vi "Test LockinEngine.vi"(8 "error in (no error)":errorcluster, 11 "Lockin.DAQ":refnum<class "Lockin.DAQ.lvclass">) -> (0 "error out":errorcluster, 3 "Lockin.DAQ":refnum<class "Lockin.DAQ.lvclass">)   [LabVIEW 2019, in "Lockin.DAQ.lvclass"]
uses:
  Lockin.DAQ.lvclass
  Typedefs/AO-cluster.ctl
  Instrument.Lockinl.UI/Typedefs/AO Channel--Cluster.ctl
  Typedefs/Function-enum.ctl
  Waveguide Model/Waveguide Model--Cluster.ctl
  Instrument.Lockin/Typedefs/Results Type--Enum.ctl
  Typedefs/Sampling.ctl
  Typedefs/REF-cluster.ctl
  Instrument.Lockinl.UI/Typedefs/REF Channel--Cluster.ctl
  Lockin.DAQ.lvclass/Lockin.DAQ.ctl
  <vilib>/Analysis/baseanly.llb/Mean (DBL).vi
  <vilib>/Analysis/NI_AALBase.lvlib
  Instrument.Lockin/Instrument.Lockin.lvclass
  Instrument.Lockinl.UI/Instrument.Lockin.UI.lvclass
panel:
  in  "Configuration.Channels: REF":T1 {"Order" min=1; "TC" min=0.0001 format="%#_3p"; "Phase" format="%.3g"; "Frequency" min=0.0001 max=10000.0 format="%.3g"}
  out "refresh rate (Hz)":dbl
  out "Waveform Graph":dbl[][](graph)
  in  "buffer size (samples)":i32
  in  "intervals":i32=10
  out "Histogram Graph":T3(graph)
  in  "sampling":T4={"Fs"=204789.0, "#s"=15753}
  in  "Type":T5
  in  "stop":bool
  in  "Simulate Waveguide":bool
  out "Average time (ms)":dbl=0.328125
  in  "Waveguide Cluster":T6
  out "Waveform Chart 2":u32(graph)
  out "Waveform Chart":dbl[][](graph)=[[-0.22911635604378638]]
  in  "AO Chanels":T7=[{"Enable?"=FALSE, "Channel"=0, "Amplitude"=0.0, "Offset"=0.0, "Frequency"=0.1, "Phase"=0.0, "Function"=enum."Sine", "Sweeping?"=FALSE}] {"Phase" format="%.3g"; "Frequency" min=0.0001 max=10000.0 format="%.3g"; "Offset" format="%.3p"; "Amplitude" min=0.0 max=10.0 format="%.3p"}
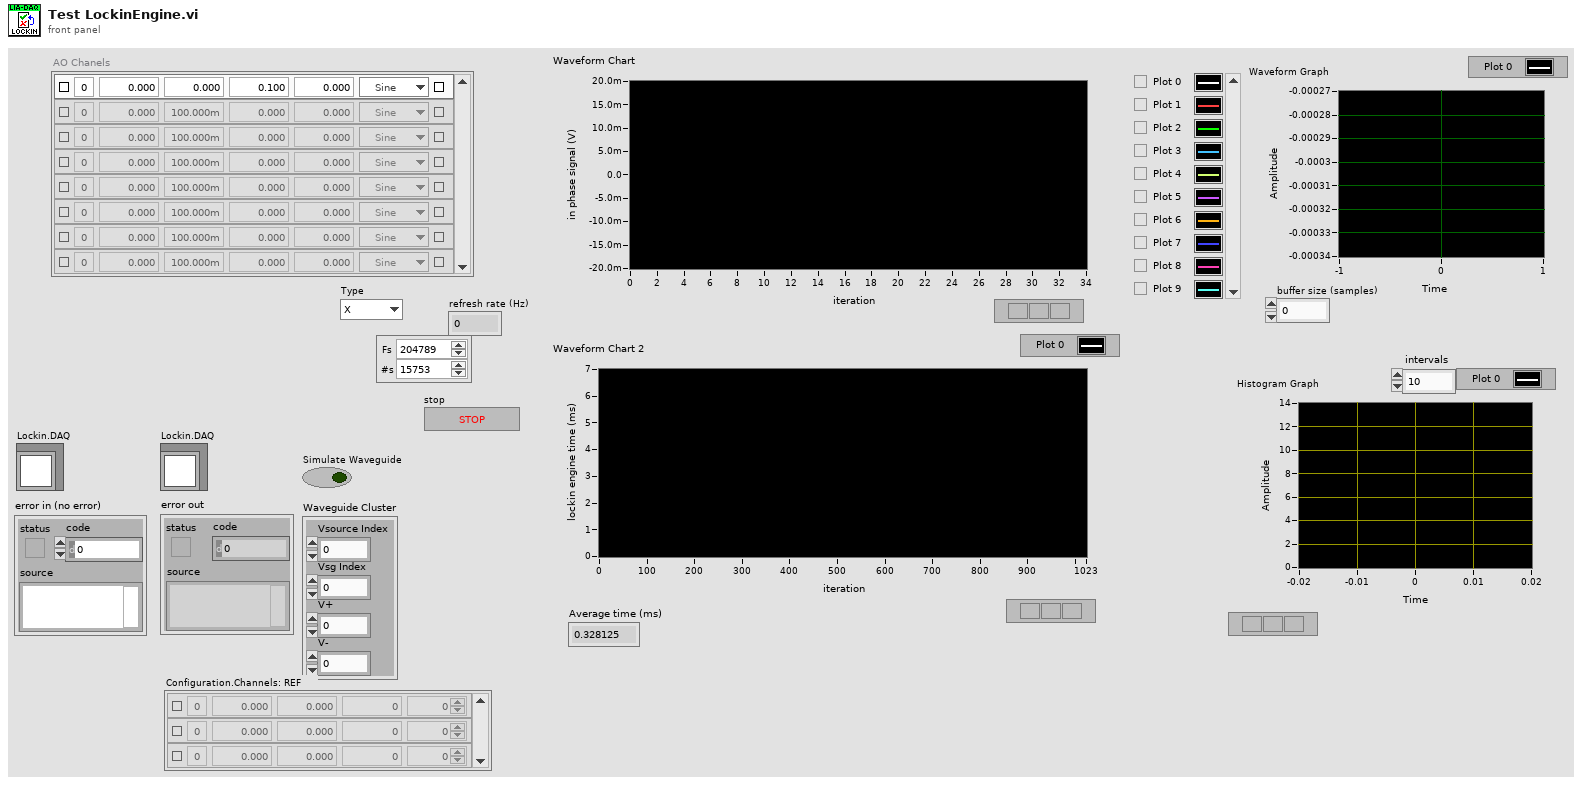
[diagram p1: front panel]
types:
  T1 = typedef "Lockin.DAQ.lvclass/REF-cluster.ctl" = T2[]
  T2 = typedef "Instrument.Lockin.UI.lvclass/REF Channel--Cluster.ctl" = cluster{"Enable?":bool, "Channel":i32, "Frequency":dbl, "Phase":dbl, "TC":dbl, "Order":i32}
  T3 = cluster{"X Values":dbl[], "Histogram: h(x)":i32[]}[]
  T4 = typedef "Lockin.DAQ.lvclass/Sampling.ctl" = cluster{"Fs":dbl, "#s":i32}
  T5 = typedef "Instrument.Lockin.lvclass/Results Type--Enum.ctl" = enum16{"X", "Y", "R", "Theta", "Mean"}
  T6 = typedef "Lockin.DAQ.lvclass/Waveguide Model--Cluster.ctl" = cluster{"Vsource Index":i32, "Vsg Index":i32, "V+":i32, "V-":i32}
  T7 = typedef "Lockin.DAQ.lvclass/AO-cluster.ctl" = T8[]
  T8 = typedef "Instrument.Lockin.UI.lvclass/AO Channel--Cluster.ctl" = cluster{"Enable?":bool, "Channel":i32, "Amplitude":dbl, "Offset":dbl, "Frequency":dbl, "Phase":dbl, "Function":T9, "Sweeping?":bool}
  T9 = typedef "Lockin.DAQ.lvclass/Function-enum.ctl" = enum16{"Sine", "Triangle", "Square"}
  T10 = cluster{"X":waveform(dbl)[], "Y":waveform(dbl)[]}
  T11 = typedef "Lockin.DAQ.lvclass/Results--Cluster.ctl" = cluster{"Time Stamp":timestamp, "Results (Dictionary)":cluster{"key":string, "value":dbl}[]}
  T12 = cluster{"X Values":dbl[], "Histogram: h(x)":i32[]}
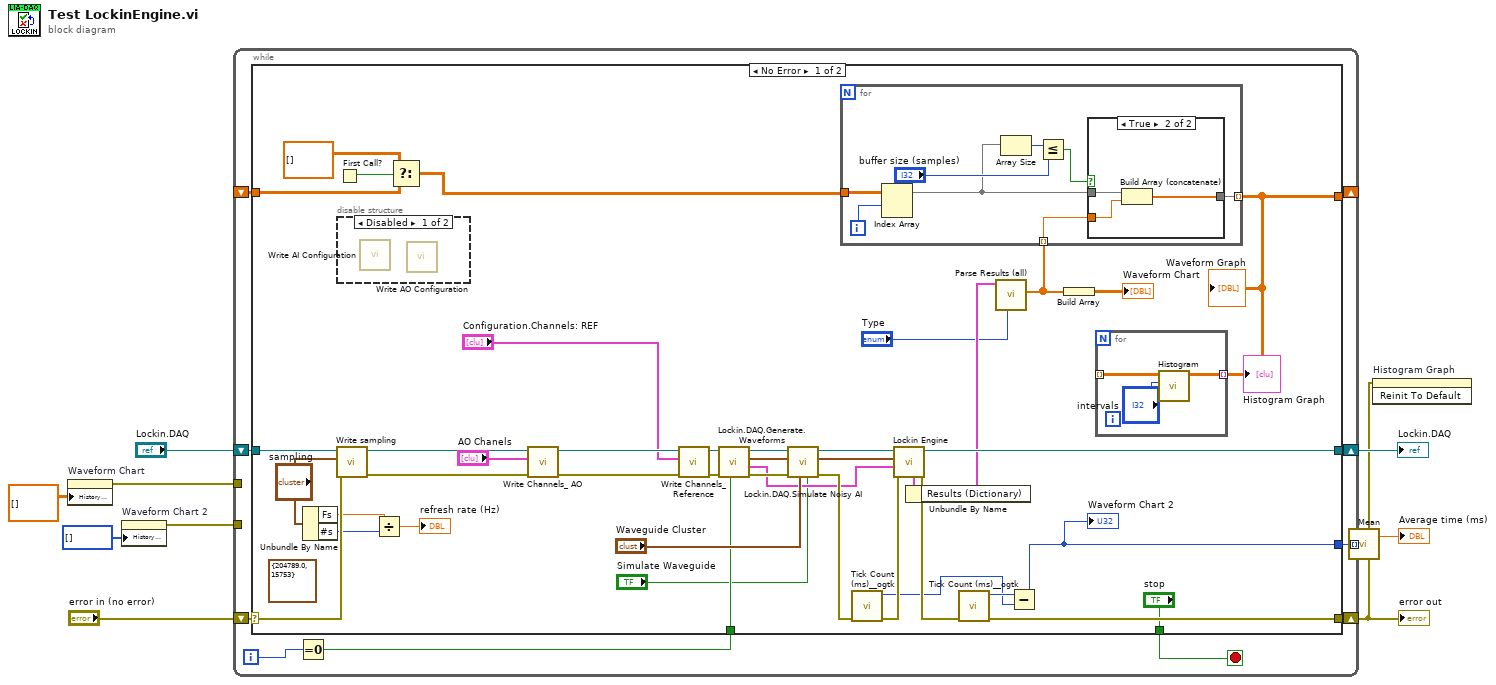
[diagram p0: block diagram]
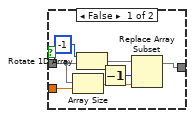
[diagram p2: hidden frame]
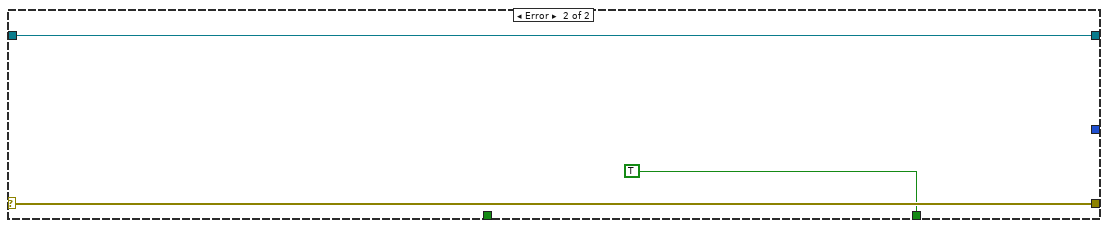
[diagram p4: hidden frame]
diagram:
  n1 = property on="Waveform Chart" class="WFChart (strict)"("History Data"=dbl[][] []) -> (error out=w3:errorcluster)  [unwired: 2 in, 1 out]
  n2 = property on="Waveform Chart 2" class="WFChart (strict)"("History Data"=u32[] []) -> (error out=w4:errorcluster)  [unwired: 2 in, 1 out]
  n3 = while {
    shift-right: [w19] -> w1
    shift-left: "error in (no error)" -> [w20]
    shift-right: [w17] -> w8
    shift-left: "Lockin.DAQ" -> [w18]
    tunnel: [w16] -> w5 mode=indexing
    tunnel: w4 -> [_]
    tunnel: w3 -> [_]
    shift-right: [w12] -> _
    shift-left: _ -> [w11]
    i -> [w14]
    stop <- w13 stop-if-true
    n4 = Equal To 0?(x=w14) -> (x = 0?=w15:bool)
    n5 = case shown="No Error" w20 {
      selector: w20 -> [w59 w87]
      tunnel: [w47 w87] -> w19
      tunnel: [w56 w86] -> w17
      tunnel: w18 -> [w60 w86]
      tunnel: [w45 _] -> w16
      tunnel: w15 -> [w41 _]
      tunnel: ["stop" TRUE ("stop")] -> w13
      tunnel: [w34 _] -> w12
      tunnel: w11 -> [w29 _]
      frame No Error {
        (unwired) T4 {"Fs"=204789.0, "#s"=15753} ("sampling")
        n6 = Unbundle By Name("sampling") -> ("Fs"=w27:dbl, "#s"=w26:i32)
        n7 = First Call?() -> (First Call?: T/F=w31:bool)
        n8 = call "Write sampling.vi"("error in (no error)"=w59, "sampling"="sampling", "Lockin.DAQ"=w60) -> ("error out"=w52:errorcluster, "Lockin.DAQ out"=w53:refnum<class "Lockin.DAQ.lvclass">)  [unwired: 7 in]
        n9 = disable-structure shown="Disabled" {
          frame Disabled {
            n10 = call "Write AI Configuration.vi"() -> ()  [unwired: 10 in, 2 out]
            n11 = call "Write AO Configuration.vi"() -> ()  [unwired: 10 in, 2 out]
          }
          frame Enabled {
          }
        }
        n12 = Divide(x=w27, y=w26) -> (x/y=→"refresh rate (Hz)":dbl)
        n13 = Select(t=dbl[][] [], s=w31, f=w29) -> (s? t:f=w30:dbl[][])
        n14 = call "Write Channels_ AO.vi"("error in (no error)"=w52, "Channels: AO"="AO Chanels", "Lockin.DAQ"=w53) -> ("error out"=w54:errorcluster, "Lockin.DAQ out"=w55:refnum<class "Lockin.DAQ.lvclass">)  [unwired: 7 in]
        n15 = call "Write Channels_ Reference.vi"("error in (no error)"=w54, "Configuration.Channels: REF"="Configuration.Channels: REF", "Lockin.DAQ"=w55) -> ("error out"=w38:errorcluster, "Lockin.DAQ out"=w37:refnum<class "Lockin.DAQ.lvclass">)  [unwired: 7 in]
        n16 = call "Lockin.DAQ.Generate.Waveforms.vi"("Reset Phase?"=w41, "error in (no error)"=w38, "Lockin.DAQ"=w37) -> ("error out"=w61:errorcluster, "Reference"=w40:T10, "AO []"=w63:waveform(dbl)[], "Lockin.DAQ"=w62:refnum<class "Lockin.DAQ.lvclass">)  [unwired: 5 in]
        n17 = call "Lockin.DAQ.Simulate Noisy AI.vi"("Simulate Waveguide [T]"="Simulate Waveguide", "Waveguide Cluster"="Waveguide Cluster", "error in (no error)"=w61, "AO []"=w63, "Lockin.DAQ in"=w62) -> ("error out"=w49:errorcluster, "Noisy AI []"=w58:waveform(dbl)[], "Lockin.DAQ out"=w57:refnum<class "Lockin.DAQ.lvclass">)  [unwired: 4 in]
        n18 = call <userlib>:"Tick Count (ms)__ogtk.vi"("error in (no error)"=w49) -> ("error out"=w48:errorcluster, "millisecond timer value"=w35:u32)  [unwired: 9 in]
        n19 = call "Lockin Engine.vi"("error in (no error)"=w48, "Reference"=w40, "AI Waveforms"=w58, "Lockin.DAQ"=w57) -> ("error out"=w44:errorcluster, "Averaged Results (X,Y,R,Theta,Mean)"=w50:T11, "Lockin.DAQ"=w56:refnum<class "Lockin.DAQ.lvclass">)  [unwired: 4 in, 1 out]
        n20 = Unbundle By Name(w50) -> ("Results (Dictionary)"=w23:cluster{"key":string, "value":dbl}[])
        n21 = call <userlib>:"Tick Count (ms)__ogtk.vi"("error in (no error)"=w44) -> ("error out"=w47:errorcluster, "millisecond timer value"=w46:u32)  [unwired: 9 in]
        n22 = call "Parse Results (all).vi"("Type"="Type", "Results (Dictionary)"=w23) -> ("Data"=w22:dbl[])  [unwired: 6 in, 3 out]
        n23 = for {
          tunnel: w30 -> [w74]
          tunnel: [w70] -> w34 mode=indexing
          tunnel: w22 -> [w69] mode=indexing
          i -> [w67]
          n24 = Index Array(array=w74, index (row)=w67) -> (element=w68:dbl[])  [unwired: 1 in]
          n25 = Array Size(array=w68) -> (size(s)=w73:i32)
          n26 = Less Or Equal?(x=w73, y="buffer size (samples)") -> (x <= y?=w71:bool)
          n27 = case shown="True" w71 {
            tunnel: [w76 w84] -> w70
            tunnel: w69 -> [w79 w82]
            tunnel: w68 -> [w78 w83]
            frame False {
              n28 = Array Size(array=w78) -> (size(s)=w77:i32)
              n29 = Rotate 1D Array(1:w78, 2:-1 ("n")) -> (0:w80:dbl[])
              n30 = Decrement(x=w77) -> (x-1=w75:i32)
              n31 = Replace Array Subset(array=w80, new element=w79, index=w75) -> (w76:dbl[])
            }
            frame True {
              n32 = Build Array (concatenate)(w83, w82) -> (w84:dbl[])
            }
          }
        }
        "Waveform Graph" <- w34
        n33 = Subtract(x=w46, y=w35) -> (x-y=w45:u32)
        "Waveform Chart 2" <- w45
        n34 = Build Array(w22) -> (→"Waveform Chart":dbl[][])
        n35 = for {
          tunnel: w34 -> [w65] mode=indexing
          tunnel: [w64] -> w33 mode=indexing
          n36 = call <vilib>:"Histogram.vi"("intervals"="intervals", "X"=w65) -> ("Histogram Graph"=w64:T12)  [unwired: 6 in, 3 out]
        }
        "Histogram Graph" <- w33
      }
      frame Error {
      }
    }
  }
  "error out" <- w1
  "Lockin.DAQ" <- w8
  n37 = call-poly <vilib>:"Mean.vi"("X"=w5) -> ("mean"=→"Average time (ms)":dbl)  [unwired: 1 out]
  n38 = invoke on="Histogram Graph" class="XYGraph (strict)" method="Reinit To Default"(error in=w1) -> ()  [unwired: 2 in, 3 out]
